vi "StahlPS_Pbus.UpdateCurrent.vi"(0 "i ref in":refnum<vi>, 1 "badValue":bool, 2 "moduleValue":dbl format="%.2f", 3 "ms timeout (10000)":i32=10000, 5 "error in (no error)":errorcluster, 6 "quality":i32) -> (14 "i ref out":refnum<vi>, 17 "timed out":bool, 19 "error out":errorcluster)   [LabVIEW 2014, in "StahlPS_Pbus.lvlib"]
doc: "Takes the inpute (raw) voltage and calcutes the real actual current [A] delivered by the power supply.\n\nThe value of the actual current is written to the attribute data and published via DIM.\n\nThe bad-status bit is also determined and updated."
uses:
  StahlPS_Pbus.lvlib
  CSlibraries/UtilityLib/UtilityLib.valueStatus.ctl
  CSCore/CSApplicationBaseClasses/PSChannelBase/PSChannelBase.directionType.ctl
  CSCore/CSApplicationBaseClasses/PSChannelBase/PSChannelBase.serviceType.ctl
  CSCore/CSApplicationBaseClasses/DeviceBase/DeviceBase.deviceState.ctl
  CSCore/CSApplicationBaseClasses/PSChannelBase/PSChannelBase.lvlib
  CSlibraries/UtilityLib/UtilityLib.lvlib
  CSCore/CSApplicationBaseClasses/DeviceBase/DeviceBase.lvlib
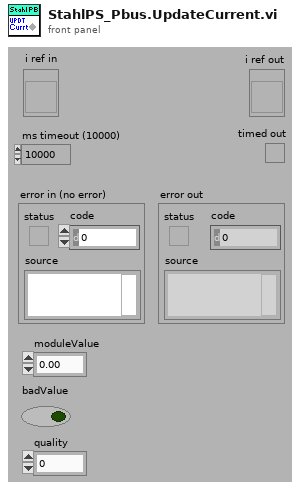
[diagram p1: front panel]
types:
  T1 = typedef "PSChannelBase.lvlib/PSChannelBase.serviceType.ctl" = enum16{"onOff", "voltage", "current", "tripCurrent", "rampUpSpeed", "rampDownSpeed", "status"}
  T2 = typedef "PSChannelBase.lvlib/PSChannelBase.directionType.ctl" = enum16{"unknown", "update actual value", "update nominal value", "update both"}
  T3 = typedef "UtilityLib.lvlib/UtilityLib.valueStatus.ctl" = enum16{"no info available", "stand by/off", "on", "warning", "alarm/malfunction", "not implemented", "user action required", "important information", "system default", "control default", "indicator default", "button default"}
  T4 = typedef "DeviceBase.lvlib/DeviceBase.deviceState.ctl" = i16
  T5 = typedef "StahlPS_Pbus.lvlib/StahlPS_Pbus.i attribute.ctl" = cluster{"Type":string, "CALC_FACTOR_SET_VOLTAGE":dbl, "CALC_FACTOR_GET_VOLTAGE":dbl, "CALC_FACTOR_GET_CURRENT":dbl, "CALC_FACTOR_SET_CURRENT ":dbl, "REG_VALUE":dbl, "Sign":bool, "setVoltIDs":i32[], "Elektrode Names":string[]}
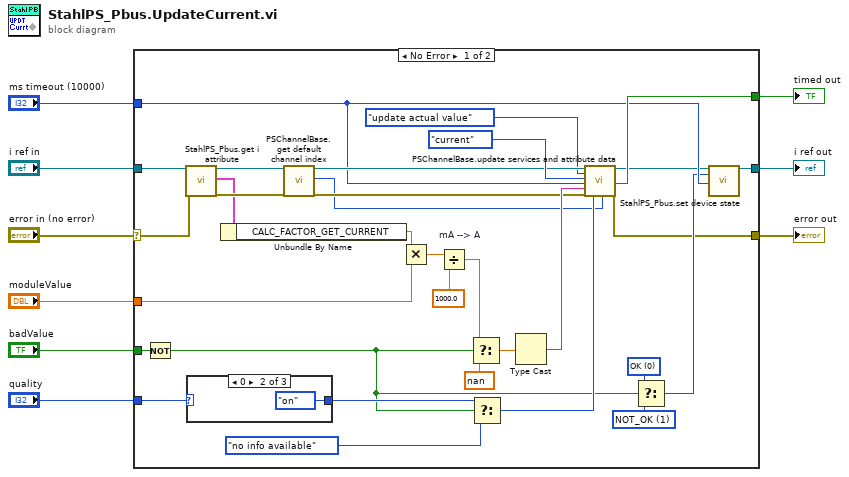
[diagram p0: block diagram]
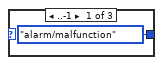
[diagram p2: hidden frame]
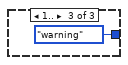
[diagram p3: hidden frame]
diagram:
  n1 = case shown="No Error" "error in (no error)" {
    selector: "error in (no error)" -> [w29 w45]
    tunnel: "i ref in" -> [w30 w46]
    tunnel: "moduleValue" -> [w25 _]
    tunnel: "ms timeout (10000)" -> [w17 _]
    tunnel: [w12 w46] -> w6
    tunnel: [w10 w45] -> w5
    tunnel: [w20 _] -> w4
    tunnel: "badValue" -> [w41 _]
    tunnel: "quality" -> [w40 _]
    frame No Error {
      w14 = T4 1 items=["ERROR"=-1, "OK"=0, "NOT_OK"=1] ("f")
      w15 = T4 0 items=["ERROR"=-1, "OK"=0, "NOT_OK"=1] ("deviceState")
      n2 = Not(x=w41) -> (.not. x?=w16:bool)
      n3 = call "StahlPS_Pbus.get i attribute.vi"("i ref in"=w30, "error in (no error)"=w29) -> ("i ref out"=w28:refnum<vi>, "i attribute"=w26:T5, "error out"=w27:errorcluster)  [unwired: 15 in]
      n4 = case shown="0" w40 {
        tunnel: [UtilityLib.valueStatus."alarm/malfunction" ("quality") UtilityLib.valueStatus."on" ("quality") UtilityLib.valueStatus."warning" ("quality")] -> w39
        frame ..-1 {
        }
        frame 0 {
        }
        frame 1.. {
        }
      }
      n5 = Unbundle By Name(w26) -> ("CALC_FACTOR_GET_CURRENT"=w31:dbl)
      n6 = call "PSChannelBase.get default channel index.vi"("i ref in"=w28, "error in (no error)"=w27) -> ("i ref out"=w34:refnum<vi>, "defaultChannelIndex"=w19:i32, "error out"=w33:errorcluster)  [unwired: 15 in]
      n7 = Multiply(x=w31, y=w25) -> (x*y=w23:dbl)
      n8 = Divide "mA --> A"(x=w23, y=1000.0) -> (x/y=w22:dbl)
      n9 = Select(t=w22, s=w16, f=nan) -> (s? t:f=w36:dbl)
      n10 = Select(t=w39, s=w16, f=UtilityLib.valueStatus."no info available" ("quality")) -> (s? t:f=w32:T3)
      n11 = Type Cast(x=w36) -> (*(type *) &x=w35:string)  [unwired: 1 in]
      n12 = call "PSChannelBase.update services and attribute data.vi"("i ref in"=w34, "direction"=PSChannelBase.directionType."update actual value", "service"=PSChannelBase.serviceType."current", "ms timeout (10000)"=w17, "value"=w35, "error in (no error)"=w33, "quality"=w32, "channelNumber"=w19) -> ("i ref out"=w11:refnum<vi>, "timed out"=w20:bool, "error out"=w10:errorcluster)  [unwired: 9 in]
      n13 = Select(t=w15, s=w16, f=w14) -> (s? t:f=w13:T4)
      n14 = call "StahlPS_Pbus.set device state.vi"("i ref in"=w11, "deviceState"=w13, "ms timeout (10000)"=w17) -> ("i ref out"=w12:refnum<vi>)  [unwired: 14 in, 2 out]
    }
    frame Error {
    }
  }
  "error out" <- w5
  "i ref out" <- w6
  "timed out" <- w4
